vi "Measurement Parser.vi"(7 "Waveform Graph":dynamicdata(graph), 8 "error in (no error)":errorcluster, 9 "Generic Card in":refnum<class "Generic Card.lvclass">, 10 "Data Array":dbl[](array[numeric]), 11 "Abstract Sensor in":refnum<class "Abstract Sensor.lvclass">) -> (0 "error out":errorcluster, 3 "Abstract Sensor out":refnum<class "Abstract Sensor.lvclass">)   [LabVIEW 2016, in "Abstract Sensor.lvlib" / "Abstract Sensor.lvclass"]
uses:
  Abstract Sensor.lvclass
  Generic Instrument/Generic Card/Generic Card.lvclass
panel:
  out "Waveform Graph 2":dbl
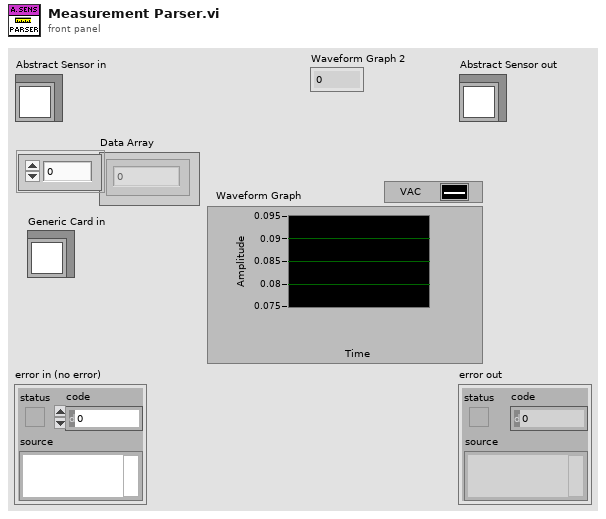
[diagram p1: front panel]
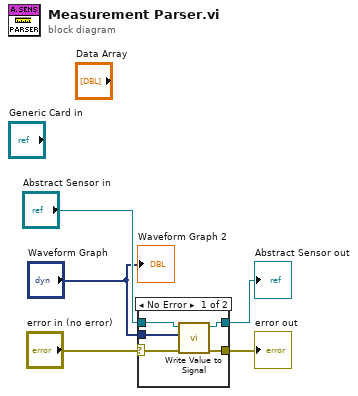
[diagram p0: block diagram]
diagram:
  n1 = case shown="No Error" "error in (no error)" {
    selector: "error in (no error)" -> [w8 w12]
    tunnel: [w7 w12] -> w4
    tunnel: [w9 w11] -> w2
    tunnel: "Abstract Sensor in" -> [w10 w11]
    tunnel: "Waveform Graph" -> [w6 _]
    frame No Error {
      n2 = call-dynamic "Write Value to Signal.vi"("error in (no error)"=w8, "Waveform Graph"=w6, "Abstract Sensor in"=w10) -> ("error out"=w7:errorcluster, "Abstract Sensor out"=w9:refnum<class "Abstract Sensor.lvclass">)  [unwired: 7 in]
    }
    frame Error {
    }
  }
  "error out" <- w4
  "Abstract Sensor out" <- w2
  "Waveform Graph 2" <- "Waveform Graph"
